vi "ODE substitute parameters.vi"(3 "Formula String Parameters":T1, 4 "parameters":string[](array[string]), 5 "values":dbl[](array[numeric])) -> (0 "Formula String Parameters with substitutions":T1)   [LabVIEW 2018]
doc: "Substitute parameters."
uses:
  <vilib>/gmath/NI_Gmath.lvlib
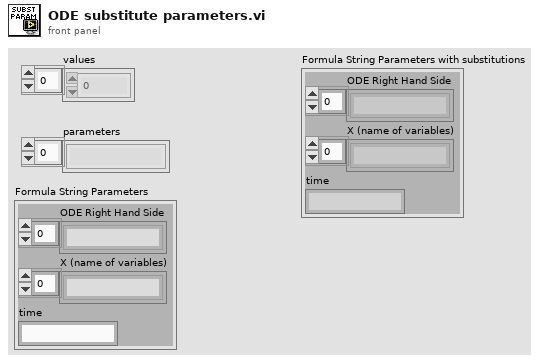
[diagram p1: front panel]
types:
  T1 = cluster{"ODE Right Hand Side":string[], "X (name of variables)":string[], "time":string}
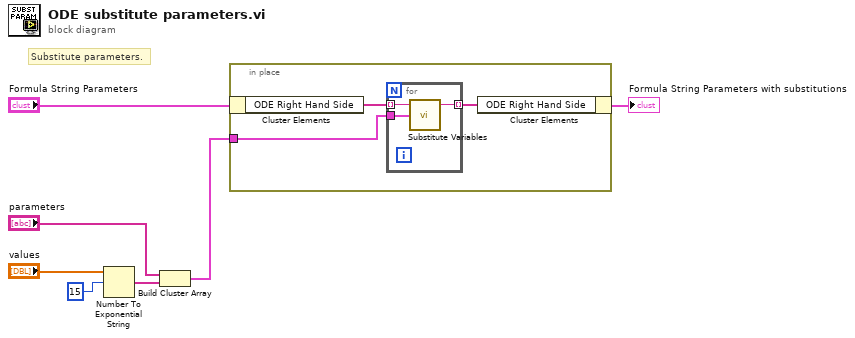
[diagram p0: block diagram]
diagram:
  # "Substitute parameters."
  n1 = Number To Exponential String(number="values", 3:i16 15 ("width (-)")) -> (E-format string=w6:string[])  [unwired: 2 out]
  n2 = Build Cluster Array("parameters", w6) -> (w7:cluster{"Bundle Element":string, "d":string}[])
  n3 = in-place {
    in-place-border: w7 -> [w9]
    n4 = in-place-cluster #1("Formula String Parameters") -> ("ODE Right Hand Side"=w8:string[])
    n5 = for {
      tunnel: w8 -> [w13] mode=indexing
      tunnel: w9 -> [w12]
      tunnel: [w11] -> w10 mode=indexing
      n6 = call <vilib>:"Substitute Variables.vi"("Substitution Rules"=w12, "original formula"=w13) -> ("formula after substitution"=w11:string)  [unwired: 1 in, 1 out]
    }
    n7 = in-place-cluster #1("ODE Right Hand Side"=w10) -> (→"Formula String Parameters with substitutions":T1)
  }
